vi "Get Message-Enqueuer Component Paths.vi"(8 "error in (no error)":errorcluster, 11 "LVClassLibrary in":refnum<vi>) -> (0 "error out":errorcluster, 2 "Paths":T1, 3 "LVClassLibrary out":refnum<vi>)   [LabVIEW 2018, in "Scripting.lvlib"]
uses:
  Scripting.lvlib
  Message-Enqueuer Component Paths.ctl
  Actor Class Items.ctl
  Error-Codes.ctl
  Convert Error from Boolean False.vi
  Bundle-Error.vi
  Error-Offset.vi
  <vilib>/Utility/error.llb/Error Cluster From Error Code.vi
  Actor.lvclass
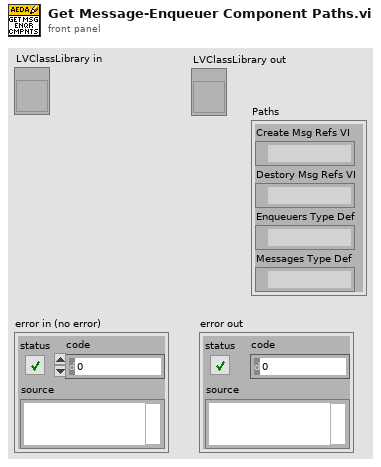
[diagram p1: front panel]
types:
  T1 = typedef "Scripting.lvlib/Message-Enqueuer Component Paths.ctl" = cluster{"Create Msg Refs VI":path, "Destory Msg Refs VI":path, "Enqueuers Type Def":path, "Messages Type Def":path}
  T2 = typedef "Scripting.lvlib/Actor.lvclass/Actor Class Items.ctl" = enum16{"Run VI", "Create Enqueuers VI", "Destroy Enqueuers VI", "Enqueuers Control", "Messages Control", "Subscribe to Broadcast"}
  T3 = typedef "Scripting.lvlib/Error-Codes.ctl" = enum16{"EVENT_REF_TYPE_DEF_IS_NESTED", "EVENT_REF_TYPE_DEF_IS_EMPTY", "EVENT_REF_TYPE_DEF_INCLUDES_NON_REFS", "EVENT_REF_TYPE_INVALID_REPLY_REF", "EVENT_REF_TYPE_REPLY_IS_NOT_TYPE_DEF", "EVENT_REF_TYPE_DEF_IS_NOT_CLUSTER", "EVENT_REF_TYPE_DEF_INVALID_REQ_REPLY_TYPE", "ACTOR_CLASS_PATH_IS_INVALID", "ACTOR_CLASS_LIBRARY_IS_NOT_EDITABLE", "ACTOR_CLASS_CREATE_ENQUEUER_REFS_VI_NOT_FOUND", "MSG_ENQUEUER_REFS_CTL_NOT_FOUND", "ACTOR_CLASS_MAIN_RUN_VI_NOT_FOUND", "ACTOR_CLASS_DESTROY_ENQUEUER_REFS_VI_NOT_FOUND", "CREATE_ENQUEUER_REFS_ERROR_TERMINAL_NOT_FOUND", "CREATE_ENQUEUER_REFS_INVALID_TYPE_DEF", "CREATE_ENQUEUER_REF_NAMEBUNDLER_NOT_FOUND", "CREATE_ENQUEUER_REF_MULTIPLE_NAMEBUNDLERS", "MESSAGES_REF_TYPE_DEF_IS_EMPTY", "MESSAGES_REF_TYPE_DEF_IS_NESTED", "ACTOR_TEMPLATE_CLASS_NOT_FOUND"}
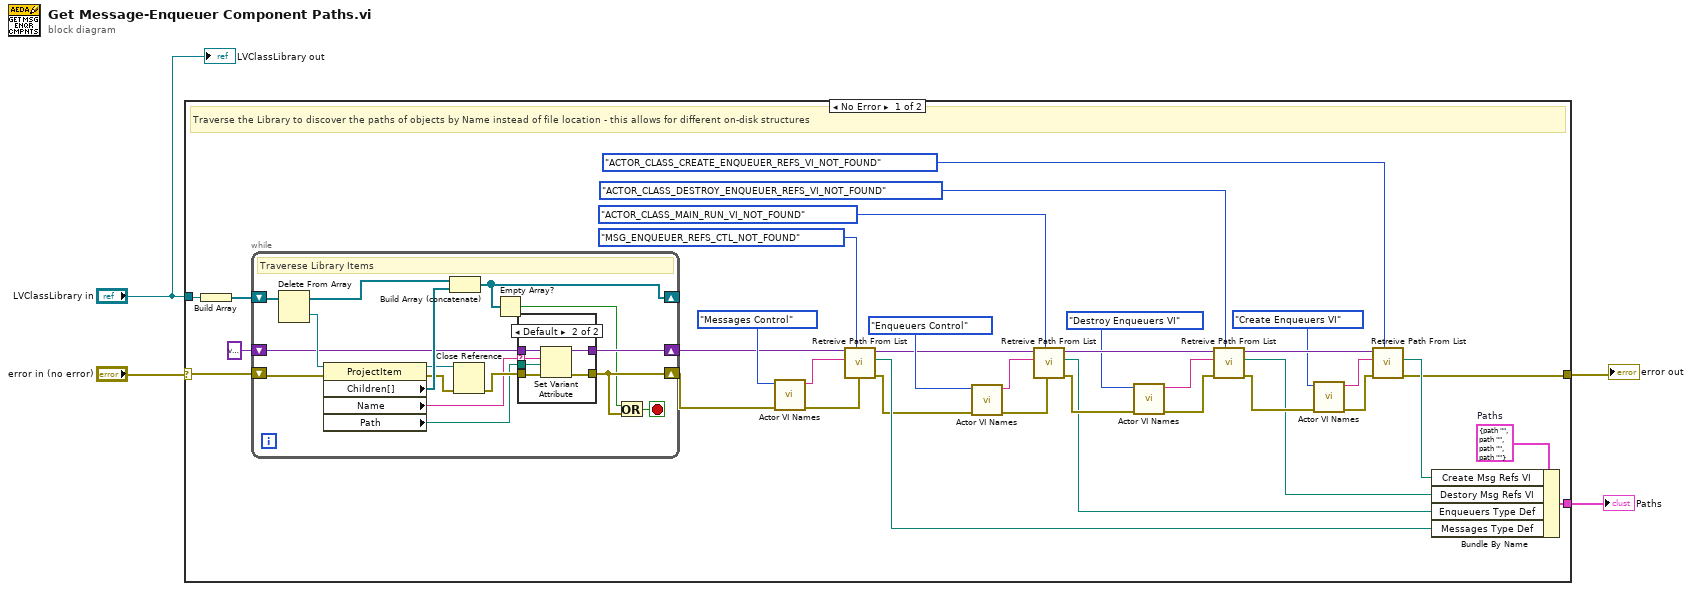
[diagram p0: block diagram]
diagram:
  n1 = case shown="No Error" "error in (no error)" {
    selector: "error in (no error)" -> [w37 w64]
    tunnel: "LVClassLibrary in" -> [w38 _]
    tunnel: [w36 _] -> w2
    tunnel: [w7 w64] -> w1
    frame No Error {
      w39 = T1 {"Create Msg Refs VI"=path "", "Destory Msg Refs VI"=path "", "Enqueuers Type Def"=path "", "Messages Type Def"=path ""}  # Paths
      # "Traverse the Library to discover the paths of objects by Name instead of file location - this allows for different on-disk structures"
      n2 = Build Array(w38) -> (w6:refnum<vi>[])
      n3 = while {
        shift-right: [w41] -> _
        shift-left: w6 -> [w55]
        shift-right: [w47] -> w30
        shift-left: variant -> [w48]
        shift-right: [w42] -> w35
        shift-left: w37 -> [w44]
        stop <- w43 stop-if-true
        # "Traverese Library Items"
        n4 = Delete From Array(array=w55) -> (deleted portion=w54:refnum<vi>, array with subset deleted=w53:refnum<vi>[])  [unwired: 2 in]
        n5 = property class="ProjectItem"(reference=w54, error in=w44) -> (reference out=w50:refnum<vi>, error out=w51:errorcluster, "Children[]"=w52:refnum<vi>[], "Name"=w46:string, "Path"=w45:path)
        n6 = Build Array (concatenate)(w53, w52) -> (w41:refnum<vi>[])
        n7 = Close Reference(reference=w50, error in (no error)=w51) -> (error out=w49:errorcluster)
        n8 = Empty Array?(array=w41) -> (empty?=w40:bool)
        n9 = case shown="Default" w46 {
          selector: w46 -> [_ w60]
          tunnel: w49 -> [w56 w63]
          tunnel: w48 -> [w57 w62]
          tunnel: [w57 w61] -> w47
          tunnel: w45 -> [_ w59]
          tunnel: [w56 w58] -> w42
          frame "" {
          }
          frame Default {
            n10 = Set Variant Attribute(Variant=w62, name=w60, value=w59, error in=w63) -> (Variant out=w61:variant, error out=w58:errorcluster)  [unwired: 1 out]
          }
        }
        n11 = Or(x=w40, y=w42) -> (x .or. y?=w43:bool)
      }
      n12 = call "Actor VI Names.vi"("error in (no error)"=w35, "Actor-Class Item"=Actor_Class_Items."Messages Control") -> ("error out"=w34:errorcluster, "Name"=w31:string)  [unwired: 8 in]
      n13 = call "Retreive Path From List.vi"("Error if Not Found"=Error-Codes."MSG_ENQUEUER_REFS_CTL_NOT_FOUND" ("Convert to Error Code"), "error in (no error)"=w34, "Name"=w31, "List in"=w30) -> ("error out"=w26:errorcluster, "Path"=w28:path, "List out"=w27:variant)  [unwired: 5 in]
      n14 = call "Actor VI Names.vi"("error in (no error)"=w26, "Actor-Class Item"=Actor_Class_Items."Enqueuers Control") -> ("error out"=w25:errorcluster, "Name"=w24:string)  [unwired: 8 in]
      n15 = call "Retreive Path From List.vi"("Error if Not Found"=Error-Codes."ACTOR_CLASS_MAIN_RUN_VI_NOT_FOUND" ("Convert to Error Code"), "error in (no error)"=w25, "Name"=w24, "List in"=w27) -> ("error out"=w21:errorcluster, "Path"=w19:path, "List out"=w22:variant)  [unwired: 5 in]
      n16 = call "Actor VI Names.vi"("error in (no error)"=w21, "Actor-Class Item"=Actor_Class_Items."Destroy Enqueuers VI") -> ("error out"=w17:errorcluster, "Name"=w18:string)  [unwired: 8 in]
      n17 = call "Retreive Path From List.vi"("Error if Not Found"=Error-Codes."ACTOR_CLASS_DESTROY_ENQUEUER_REFS_VI_NOT_FOUND" ("Convert to Error Code"), "error in (no error)"=w17, "Name"=w18, "List in"=w22) -> ("error out"=w15:errorcluster, "Path"=w12:path, "List out"=w13:variant)  [unwired: 5 in]
      n18 = call "Actor VI Names.vi"("error in (no error)"=w15, "Actor-Class Item"=Actor_Class_Items."Create Enqueuers VI") -> ("error out"=w14:errorcluster, "Name"=w10:string)  [unwired: 8 in]
      n19 = call "Retreive Path From List.vi"("Error if Not Found"=Error-Codes."ACTOR_CLASS_CREATE_ENQUEUER_REFS_VI_NOT_FOUND" ("Convert to Error Code"), "error in (no error)"=w14, "Name"=w10, "List in"=w13) -> ("error out"=w7:errorcluster, "Path"=w8:path)  [unwired: 5 in, 1 out]
      n20 = Bundle By Name(cluster=w39, "Create Msg Refs VI"=w8, "Destory Msg Refs VI"=w12, "Enqueuers Type Def"=w19, "Messages Type Def"=w28) -> (w36:T1)
    }
    frame Error {
      # "Pass Through Error"
    }
  }
  "Paths" <- w2
  "error out" <- w1
  "LVClassLibrary out" <- "LVClassLibrary in"
